vi "4Pi Obj Lock - Find Peak Position.vi"(9 "Fit Size":i32, 10 "y":dbl[](array[numeric]), 11 "x":dbl[](array[numeric])) -> (2 "Coerced Peak Position":dbl, 3 "Peak Position":dbl)   [LabVIEW 2016]
uses:
  <vilib>/Analysis/polynomials.llb/Scalar Polynomial Evaluation (DBL).vi
  <vilib>/Analysis/NI_AALPro.lvlib
panel:
  out "Fit curve":cluster{"Y":dbl[], "Y":dbl[]}[](graph)
  out "Best Polynomial Fit":dbl[](array[numeric])
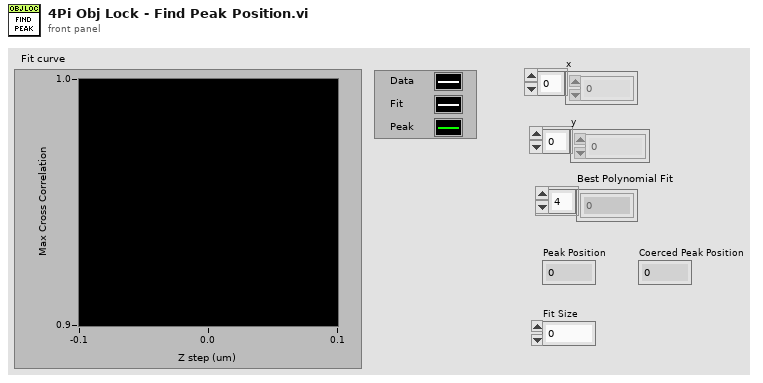
[diagram p1: front panel]
types:
  T1 = cluster{"x":dbl[], "Best Polynomial Fit":dbl[]}[]
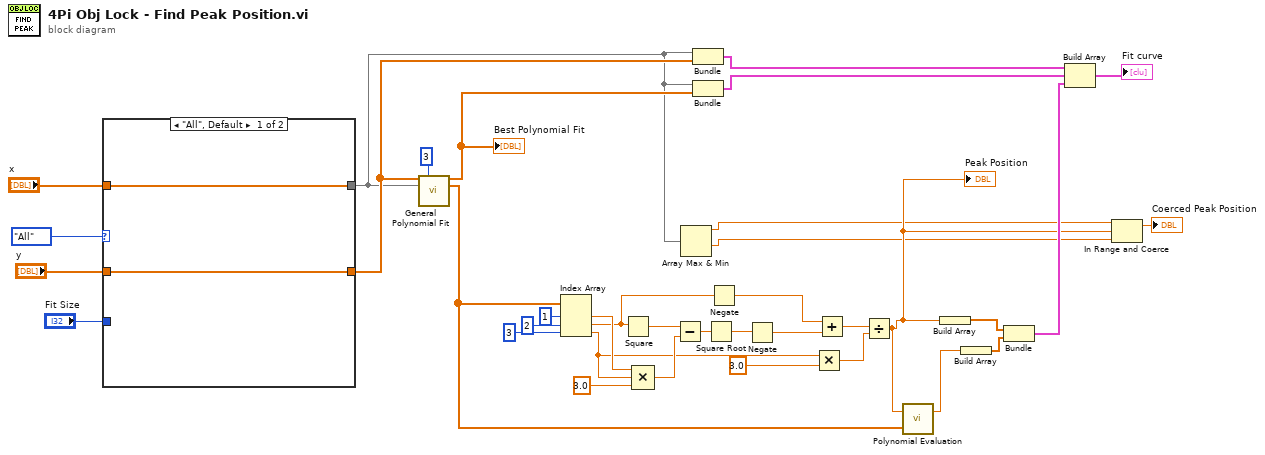
[diagram p0: block diagram]
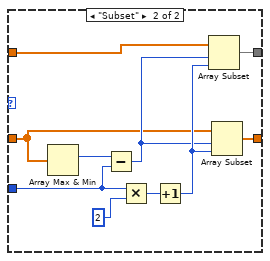
[diagram p2: hidden frame]
diagram:
  n1 = case shown="\"All\", Default" enum16{"Subset", "All"}."All" ("Enum") {
    tunnel: "x" -> [w38 w46]
    tunnel: "Fit Size" -> [_ w43]
    tunnel: "y" -> [w37 w41]
    tunnel: [w37 w40] -> w32
    tunnel: [w38 w39] -> w5
    frame "All", Default {
    }
    frame "Subset" {
      n2 = Array Max & Min(array=w41) -> (max index (indices)=w42:i32)  [unwired: 3 out]
      n3 = Subtract(x=w42, y=w43) -> (x-y=w47:i32)
      n4 = Multiply(x=w43, y=2) -> (x*y=w45:i32)
      n5 = Increment(x=w45) -> (x+1=w48:i32)
      n6 = Array Subset(array=w46, index=w47, length=w48) -> (w39:dbl[])
      n7 = Array Subset(array=w41, index=w47, length=w48) -> (w40:dbl[])
    }
  }
  n8 = call <vilib>:"General Polynomial Fit.vi"("Y"=w32, "polynomial order"=3, "X"=w5) -> ("Best Polynomial Fit"=w31:dbl[], "Polynomial Coefficients"=w8:dbl[])  [unwired: 9 in, 2 out]
  "Best Polynomial Fit" <- w31
  n9 = Index Array(array=w8, index #1=1 ("index"), index #2=2 ("index"), index #3=3 ("index")) -> (element #1=w23:dbl, element #2=w19:dbl, element #3=w16:dbl)
  n10 = Square(x=w19) -> (x^2=w24:dbl)
  n11 = Compound Arithmetic op=MULTIPLY(w23, w16, 3.0 ("value")) -> (w21:dbl)
  n12 = Subtract(x=w24, y=w21) -> (x-y=w20:dbl)
  n13 = Array Max & Min(array=w5) -> (max value=w4:dbl, min value=w3:dbl)  [unwired: 2 out]
  n14 = Bundle("x"=w5, "y"=w32) -> (w30:cluster{"x":dbl[], "y ":dbl[]})  [unwired: 1 in]
  n15 = Bundle("x"=w5, "Best Polynomial Fit"=w31) -> (w29:cluster{"x":dbl[], "Best Polynomial Fit":dbl[]})  [unwired: 1 in]
  n16 = Square Root(x=w20) -> (sqrt(x)=w10:dbl)
  n17 = Negate(x=w19) -> (-x=w18:dbl)
  n18 = Negate(x=w10) -> (-x=w9:dbl)
  n19 = Multiply(x=w16, y=3.0) -> (x*y=w14:dbl)
  n20 = Add(x=w18, y=w9) -> (x+y=w17:dbl)
  n21 = Divide(x=w17, y=w14) -> (x/y=w6:dbl)
  "Peak Position" <- w6
  n22 = call-poly <vilib>:"Polynomial Evaluation.vi"("P(x)"=w8, "a"=w6) -> ("P(a)"=w7:dbl)  [unwired: 1 out]
  n23 = Build Array(w6) -> (w13:dbl[])
  n24 = Build Array(w7) -> (w12:dbl[])
  n25 = Bundle(w13, w12) -> (w11:cluster{dbl[], dbl[]})  [unwired: 1 in]
  n26 = Build Array(w30, w29, w11) -> (→"Fit curve":T1)
  n27 = In Range and Coerce(upper limit=w4, x=w6, lower limit=w3) -> (coerced(x)=→"Coerced Peak Position":dbl)  [unwired: 1 out]
